vi "UpdateHeartRate.vi"(7 "Strict refs box":T1, 8 "error in (no error)":errorcluster, 11 "BLE Message in":refnum<class "BLE Message.lvclass">) -> (0 "error out":errorcluster, 3 "BLE Message out":refnum<class "BLE Message.lvclass">)   [LabVIEW 2015, in "BLE Message.lvclass"]
uses:
  BLE Message.lvclass
  ctrls/RefsBox.ctl
  BLE Message.lvclass/BLE Message.ctl
  <vilib>/Analysis/baseanly.llb/Mean (DBL).vi
  <vilib>/measure/mamon.llb/Waveform Peak Detection for 1 Chan.vi
  <vilib>/measure/NI_MAPro.lvlib
  <vilib>/Analysis/NI_AALBase.lvlib
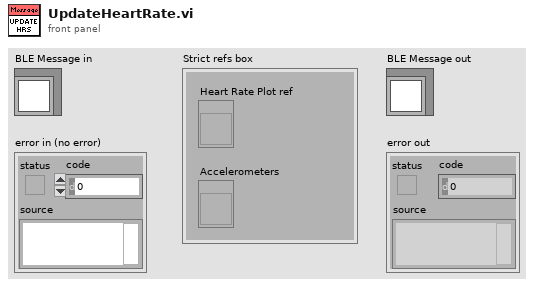
[diagram p1: front panel]
types:
  T1 = typedef "RefsBox.ctl" = cluster{"Heart Rate Plot ref":refnum<vi>, "Accelerometers":refnum<vi>}
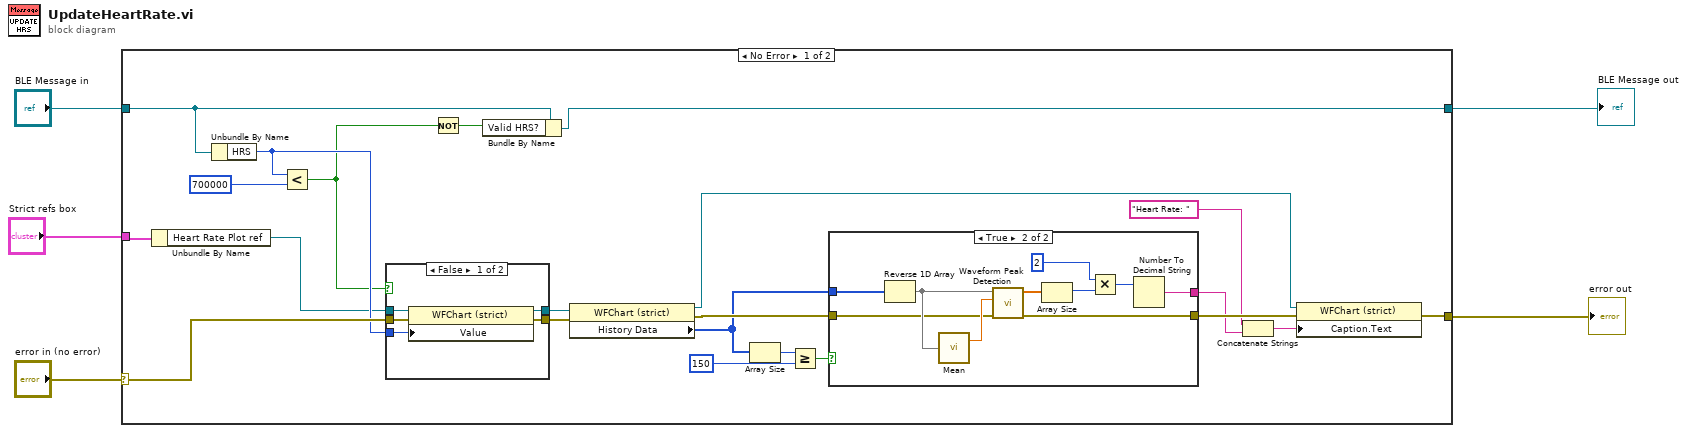
[diagram p0: block diagram]
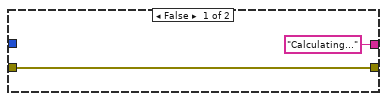
[diagram p2: hidden frame]
diagram:
  n1 = case shown="No Error" "error in (no error)" {
    selector: "error in (no error)" -> [w26 w48]
    tunnel: [w14 w48] -> w4
    tunnel: [w8 w47] -> w2
    tunnel: "BLE Message in" -> [w9 w47]
    tunnel: "Strict refs box" -> [w22 _]
    frame No Error {
      n2 = Unbundle By Name(w22) -> ("Heart Rate Plot ref"=w21:refnum<vi>)
      n3 = Unbundle By Name(w9) -> ("HRS"=w25:u32)
      n4 = Less?(x=w25, y=u32 700000) -> (x < y?=w6:bool)
      n5 = case shown="False" w6 {
        tunnel: w21 -> [w44 w45]
        tunnel: w26 -> [w43 w46]
        tunnel: w25 -> [w42 _]
        tunnel: [w41 w46] -> w24
        tunnel: [w40 w45] -> w23
        frame False {
          n6 = property class="WFChart (strict)"(reference=w44, error in=w43, "Value"=w42) -> (reference out=w40:refnum<vi>, error out=w41:errorcluster)
        }
        frame True {
        }
      }
      n7 = Not(x=w6) -> (.not. x?=w7:bool)
      n8 = Bundle By Name(cluster=w9, "Valid HRS?"=w7) -> (w8:refnum<class "BLE Message.lvclass">)
      n9 = property class="WFChart (strict)"(reference=w23, error in=w24) -> (reference out=w13:refnum<vi>, error out=w17:errorcluster, "History Data"=w16:u32[])
      n10 = Array Size(array=w16) -> (size(s)=w20:i32)
      n11 = Greater Or Equal?(x=w20, y=150) -> (x >= y?=w18:bool)
      n12 = case shown="True" w18 {
        tunnel: w17 -> [w28 w34]
        tunnel: w16 -> [_ w33]
        tunnel: ["Calculating..." w31] -> w11
        tunnel: [w28 w30] -> w15
        frame False {
        }
        frame True {
          n13 = Reverse 1D Array(array=w33) -> (reversed array=w38:u32[])
          n14 = call-poly <vilib>:"Mean.vi"("X"=w38) -> ("mean"=w39:dbl)  [unwired: 1 out]
          n15 = call-poly <vilib>:"Waveform Peak Detection.vi"("error in"=w34, "threshold"=w39, "Signal In"=w38) -> ("error out"=w30:errorcluster, "Locations"=w36:dbl[])  [unwired: 4 in, 3 out]
          n16 = Array Size(array=w36) -> (size(s)=w37:i32)
          n17 = Multiply(x=2, y=w37) -> (x*y=w32:i32)
          n18 = Number To Decimal String(number=w32) -> (decimal integer string=w31:string)  [unwired: 1 in]
        }
      }
      n19 = Concatenate Strings("Heart Rate: " ("string"), w11) -> (w12:string)
      n20 = property class="WFChart (strict)"(reference=w13, error in=w15, "Caption.Text"=w12) -> (error out=w14:errorcluster)  [unwired: 1 out]
    }
    frame Error {
    }
  }
  "error out" <- w4
  "BLE Message out" <- w2
